vi "Send Configure Triggered Voltage Level [TRG].vi"(7 "Message Priority (Normal)":T1=enum."Normal", 8 "error in (no error)":errorcluster, 9 "triggered level (0.0 Volts)":dbl format="%^.2e", 10 "channel name (\"CHANNEL1\")":string="CHANNEL1", 11 "Message Enqueuer":refnum<class "Message Enqueuer.lvclass">) -> (0 "error out":errorcluster, 3 "Message Enqueuer out":refnum<class "Message Enqueuer.lvclass">)   [LabVIEW 2013, in "CS++DCPwr.lvlib" / "Configure Triggered Voltage Level [TRG] Msg.lvclass"]
doc: "This VI sends the message to an actor."
uses:
  Configure Triggered Voltage Level [TRG] Msg.lvclass
  <vilib>/ActorFramework/Message Enqueuer/Message Enqueuer.lvclass
  <vilib>/ActorFramework/Message Enqueuer/Message Priority.ctl
  Configure Triggered Voltage Level [TRG] Msg.lvclass/Configure Triggered Voltage Level [TRG] Msg.ctl
  <vilib>/ActorFramework/Message Enqueuer/Message Enqueuer.lvclass/Message Enqueuer.ctl
  <vilib>/ActorFramework/Message Priority Queue/Priority Enqueue.vi
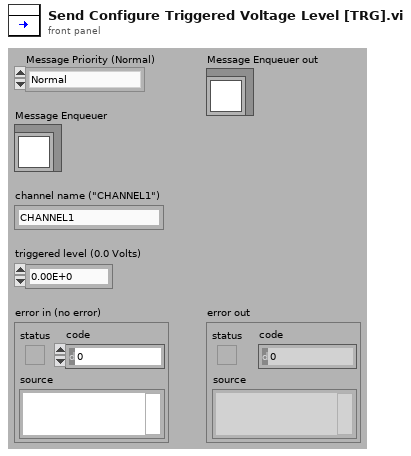
[diagram p1: front panel]
types:
  T1 = typedef "Actor Framework.lvlib/Message Enqueuer.lvclass/Message Priority.ctl" = enum16{"Low", "Normal", "High"}
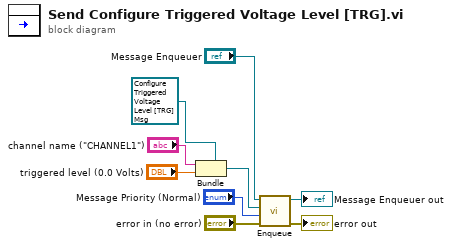
[diagram p0: block diagram]
diagram:
  n1 = Bundle(cluster=refnum<class "Configure Triggered Voltage Level [TRG] Msg.lvclass"> refnum ("Object"), "channel name (\"CHANNEL1\")", "triggered level (0.0 Volts)") -> (w5:refnum<class "Configure Triggered Voltage Level [TRG] Msg.lvclass">)
  n2 = call <vilib>:"Enqueue.vi"("error in (no error)"="error in (no error)", "Message Priority (Normal)"="Message Priority (Normal)", "Message"=w5, "Message Enqueuer in"="Message Enqueuer") -> ("error out"=→"error out":errorcluster, "Message Enqueuer out"=→"Message Enqueuer out":refnum<class "Message Enqueuer.lvclass">)  [unwired: 6 in]
